vi "读数.vi"(8 "error in":errorcluster, 11 "设置":T1) -> (0 "error out":errorcluster, 1 "响应信号":waveform(dbl)(graph) caption="采集通道", 2 "触发信号":waveform(dbl)(graph) caption="触发通道")   [LabVIEW 2018]
uses:
  <instrlib>/niScope/Configure/Trigger/niScope Configure Trigger Edge.vi
  <instrlib>/niScope/Acquire/niScope Multi Read WDT.vi
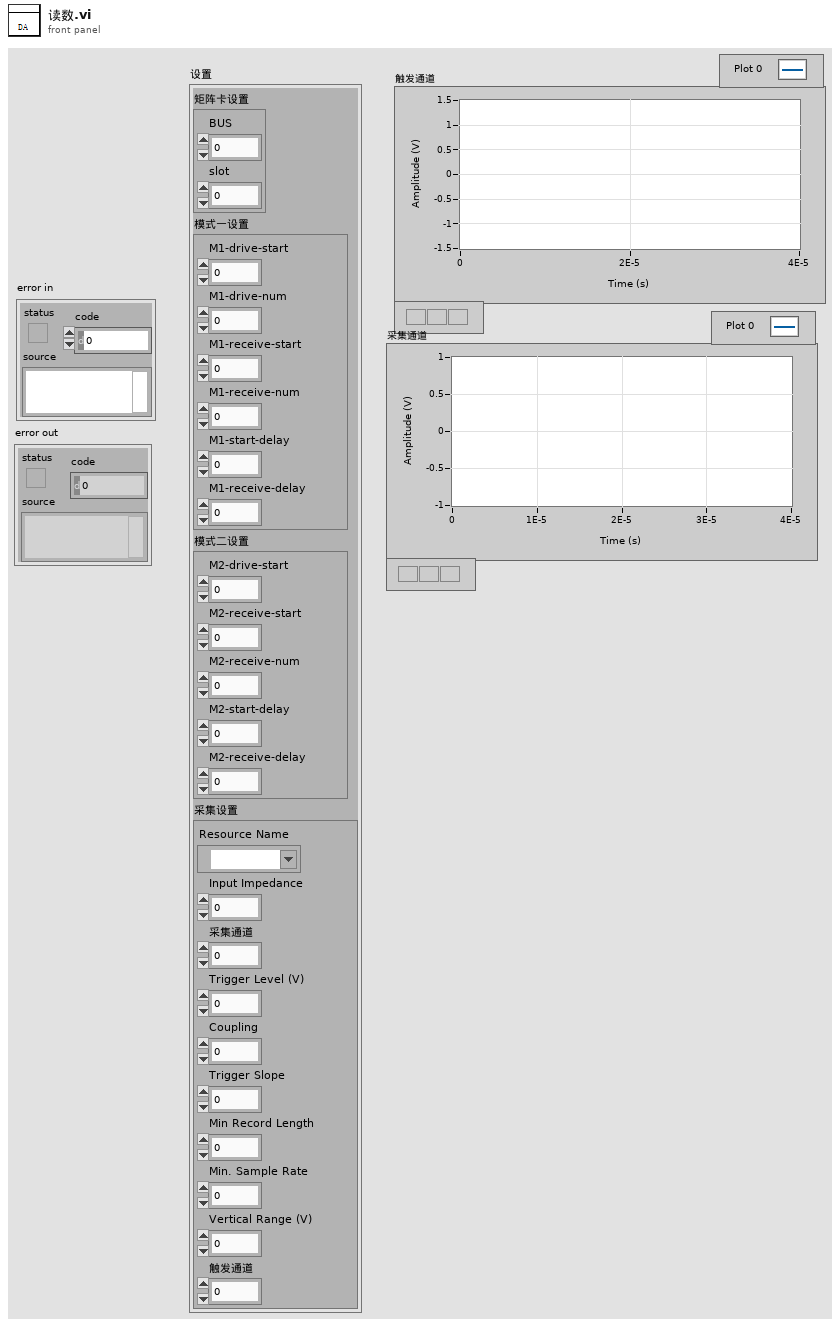
[diagram p1: front panel]
types:
  T1 = cluster{"矩阵卡设置":cluster{"BUS":u32, "slot":u32}, "模式一设置":cluster{"M1-drive-start":u32, "M1-drive-num":u32, "M1-receive-start":u32, "M1-receive-num":u32, "M1-start-delay":u32, "M1-receive-delay":u32}, "模式二设置":cluster{"M2-drive-start":u32, "M2-receive-start":u32, "M2-receive-num":u32, "M2-start-delay":u32, "M2-receive-delay":u32}, "采集设置":cluster{"Resource Name":refnum<k15>, "Input Impedance":u32, "采集通道":i32, "Trigger Level (V)":dbl, "Coupling":u16, "Trigger Slope":i32, "Min Record Length":i32, "Min. Sample Rate":dbl, "Vertical Range (V)":dbl, "触发通道":i32}}
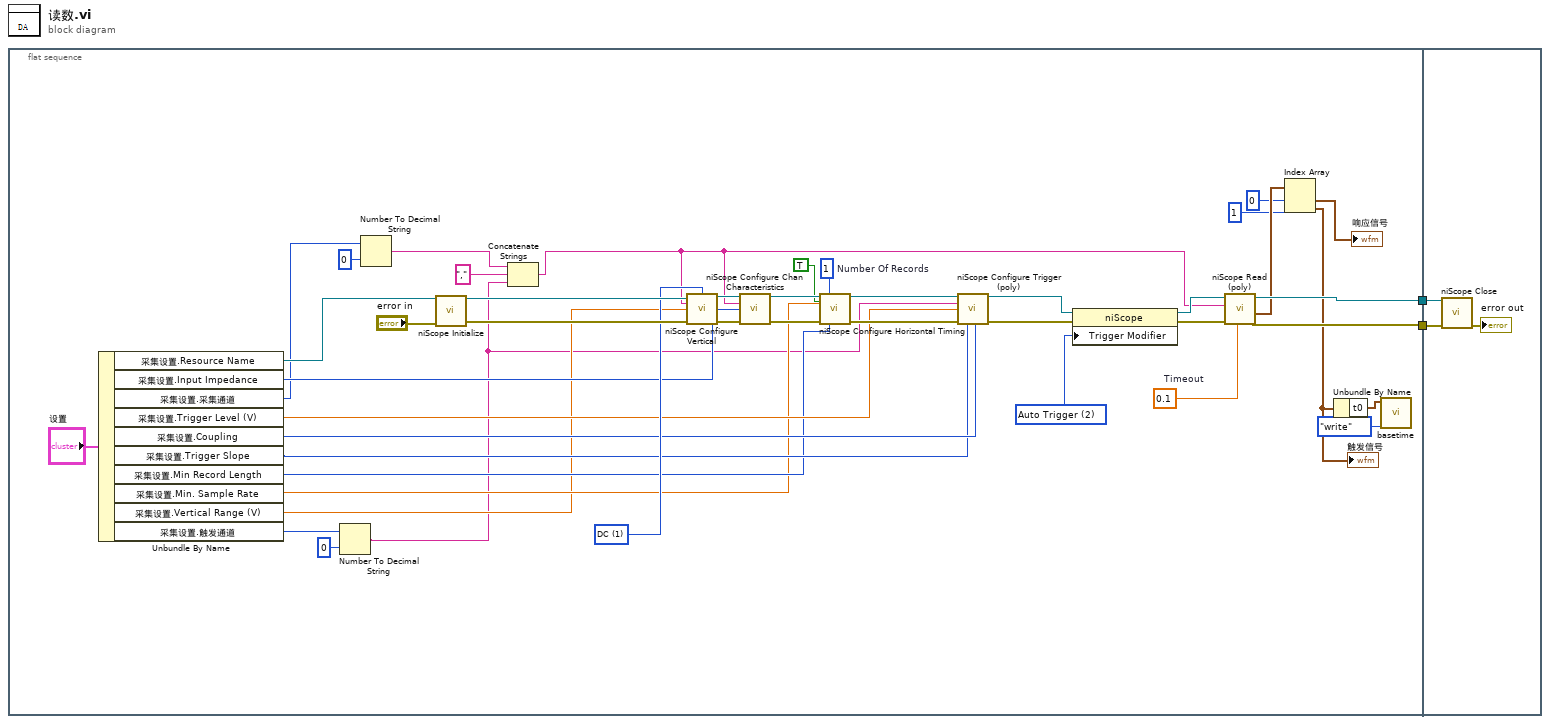
[diagram p0: block diagram]
diagram:
  n1 = flat-sequence {
    tunnel: [w11] -> w2
    tunnel: [w29] -> w1
    tunnel: w2 -> [w48]
    tunnel: w1 -> [w49]
    frame #0 {
      w30 = 1 items=["AC", "DC", "Ground"] ("Vertical Coupling")
      w31 = 2 items=["None"=1, "Auto Trigger"=2] ("Trigger Modifier")
      w34 = 1  # Number Of Records
      w32 = 0.1  # Timeout
      n2 = Unbundle By Name("设置") -> ("采集设置.Resource Name"=w28:refnum<k15>, "采集设置.Input Impedance"=w27:u32, "采集设置.采集通道"=w26:i32, "采集设置.Trigger Level (V)"=w22:dbl, "采集设置.Coupling"=w21:u16, "采集设置.Trigger Slope"=w20:i32, "采集设置.Min Record Length"=w19:i32, "采集设置.Min. Sample Rate"=w18:dbl, "采集设置.Vertical Range (V)"=w17:dbl, "采集设置.触发通道"=w23:i32)
      n3 = Number To Decimal String(number=w23, width (-)=i16 0 ("宽度(-)")) -> (decimal integer string=w5:string)
      n4 = Number To Decimal String(number=w26, width (-)=i16 0 ("宽度(-)")) -> (decimal integer string=w13:string)
      n5 = call <instrlib>:"niScope Initialize.vi"("resource name"=w28, "error in"="error in") -> ("instrument handle"=w46:refnum<k15>, "error out"=w45:errorcluster)  [unwired: 12 in]
      n6 = Concatenate Strings(w13, ",", w5) -> (w3:string)
      n7 = call <instrlib>:"niScope Configure Vertical.vi"("instrument handle"=w46, "vertical coupling"=w30, "channels"=w3, "vertical range"=w17, "error in"=w45) -> ("instrument handle out"=w37:refnum<k15>, "error out"=w38:errorcluster)  [unwired: 9 in]
      n8 = call <instrlib>:"niScope Configure Chan Characteristics.vi"("instrument handle"=w37, "channels"=w3, "input impedance"=w27, "error in"=w38) -> ("instrument handle out"=w36:refnum<k15>, "error out"=w35:errorcluster)  [unwired: 10 in]
      n9 = call <instrlib>:"niScope Configure Horizontal Timing.vi"("instrument handle"=w36, "number of records"=w34, "enforce realtime"=TRUE ("Enforce Realtime"), "min sample rate"=w18, "error in"=w35, "min record length"=w19) -> ("instrument handle out"=w43:refnum<k15>, "error out"=w44:errorcluster)  [unwired: 8 in]
      n10 = call-poly <instrlib>:"niScope Configure Trigger (poly).vi"("instrument handle"=w43, "trigger slope"=w20, "trigger coupling"=w21, "trigger source"=w5, "trigger level"=w22, "error in"=w44) -> ("instrument handle out"=w42:refnum<k15>, "error out"=w41:errorcluster)  [unwired: 8 in]
      n11 = property class="niScope"(reference=w42, error in=w41, "Trigger Modifier"=w31) -> (reference out=w39:refnum<k15>, error out=w40:errorcluster)
      n12 = call-poly <instrlib>:"niScope Read (poly).vi"("timeout"=w32, "error in"=w40, "channels"=w3, "instrument handle"=w39) -> ("error out"=w11:errorcluster, "wfm"=w10:waveform(dbl)[], "instrument handle out"=w29:refnum<k15>)  [unwired: 4 in, 1 out]
      n13 = Index Array(array=w10, index #1=0 ("索引"), index #2=1 ("索引")) -> (element #1=→"响应信号":waveform(dbl), element #2=w6:waveform(dbl))
      "触发信号" <- w6
      n14 = Unbundle By Name(w6) -> ("t0"=w4:timestamp)
      n15 = call "basetime.vi"("枚举"=enum16{"write", "read"}."write", "basetime"=w4) -> ()  [unwired: 9 in, 1 out]
    }
    frame #1 {
      n16 = call <instrlib>:"niScope Close.vi"("instrument handle"=w49, "error in"=w48) -> ("error out"=→"error out":errorcluster)  [unwired: 13 in]
    }
  }
